vi "Enqueue Q2.vi"(7 "Q1 Message":T1, 8 "error in (no error)":errorcluster, 11 "Queue Ref":T2) -> (0 "error out":errorcluster, 1 "Q2array-2D":refnum<queue>, 2 "Q2array-1D":refnum<queue>, 3 "Q2scalar":refnum<queue>)   [LabVIEW 2014]
doc: "<B>Copyright</B>: (c) MHWirth 2015. All rights reserved.\n\nAt the begining of recording, this sub VI initializes Q2 queues with Initialize 1."
uses:
  TypeDef/Q1 Message.ctl
  Data logger Scalar Enqueue Function.vi
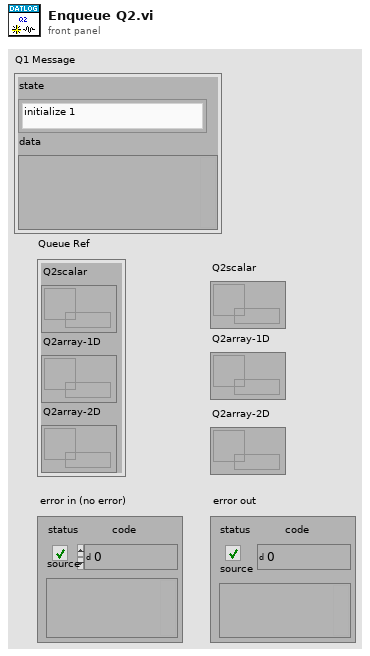
[diagram p1: front panel]
types:
  T1 = typedef "Q1 Message.ctl" = cluster{"state":enum16{"initialize 1", "initialize 2", "initialize 3", "initialize 4", "initialize 5", "initialize 6", "initialize 7", "initialize 8", "initialize 9", "Idle", "Preparation 1", "Preparation 2", "Preparation 3", "Preparation 4", "Record", "Stop recording", "Exit", "Defrag", "View", "Create Database", "Update folder setting", "Update Preference", "Update TDMS properties", "CSV Delimiter", "DB Type", "Hidden Processes", "Replace Database", "Logged File Viewer", "Defrag Prompt File", "View Prompt File", "Save to config file", "Open from config file"}, "data":variant}
  T2 = cluster{"Q2scalar":refnum<queue>, "Q2array-1D":refnum<queue>, "Q2array-2D":refnum<queue>}
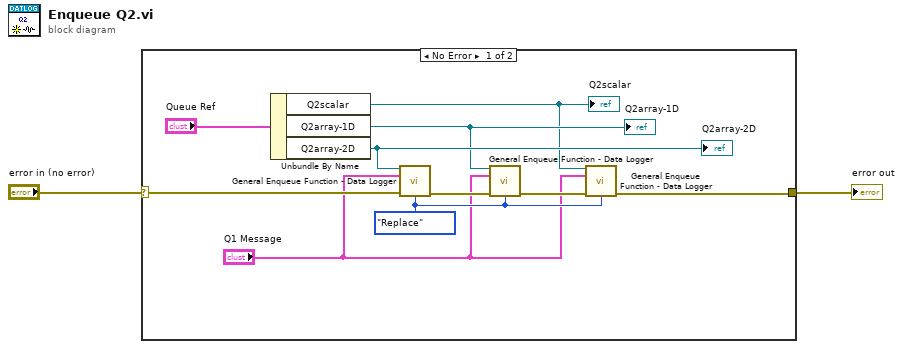
[diagram p0: block diagram]
diagram:
  n1 = case shown="No Error" "error in (no error)" {
    selector: "error in (no error)" -> [w10 w13]
    tunnel: [w3 w13] -> w1
    frame No Error {
      w5 = enum16{"Back", "Front", "Replace"}."Replace" ("Mode")
      n2 = Unbundle By Name("Queue Ref") -> ("Q2scalar"=w6:refnum<queue>, "Q2array-1D"=w8:refnum<queue>, "Q2array-2D"=w11:refnum<queue>)
      "Q2scalar" <- w6
      "Q2array-1D" <- w8
      "Q2array-2D" <- w11
      n3 = call-poly "General Enqueue Function - Data Logger.vi"("QRef in"=w11, "Q1 Message"="Q1 Message", "Error in"=w10, "Mode"=w5) -> ("Error out"=w9:errorcluster)  [unwired: 10 in, 1 out]
      n4 = call-poly "General Enqueue Function - Data Logger.vi"("QRef in"=w8, "Q1 Message"="Q1 Message", "Error in"=w9, "Mode"=w5) -> ("Error out"=w7:errorcluster)  [unwired: 10 in, 1 out]
      n5 = call-poly "General Enqueue Function - Data Logger.vi"("QRef in"=w6, "Q1 Message"="Q1 Message", "Error in"=w7, "Mode"=w5) -> ("Error out"=w3:errorcluster)  [unwired: 10 in, 1 out]
    }
    frame Error {
    }
  }
  "error out" <- w1
